vi "CalcDialogPanelBounds.vi"(8 "error in (no error)":errorcluster, 9 "Height":i32, 10 "Width":i32, 11 "Montior":i32) -> (0 "error out":errorcluster, 3 "Front Panel Window:Panel Bounds":T1)   [LabVIEW 2020, in "DP_WebView.lvclass"]
doc: "This utility will fit (resize and center) a VI (defined by the \"VI Ref\" input) about the all of the Front Panel object. It will add a border defined by border spacing in units of pixels. If no VI Reference is passed in, it will operate on the calling VI."
uses:
  DP_WebView.lvclass
  <vilib>/Utility/miscctls.llb/LVRectTypeDef.ctl
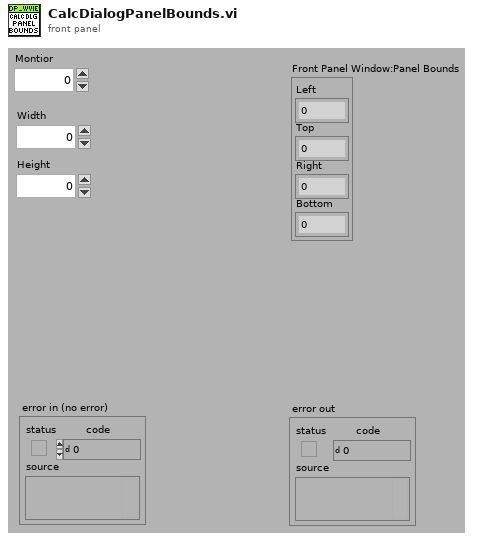
[diagram p1: front panel]
types:
  T1 = typedef "LVRectTypeDef.ctl" = cluster{"Left":i16, "Top":i16, "Right":i16, "Bottom":i16}
  T2 = typedef "LVAllMonitorsDisplayTypeDef.ctl" = cluster{"Bounds":cluster{"Left":i16, "Top":i16, "Right":i16, "Bottom":i16}, "Depth":i16}[]
  T3 = cluster{"Bounds":cluster{"Left":i16, "Top":i16, "Right":i16, "Bottom":i16}, "Depth":i16}
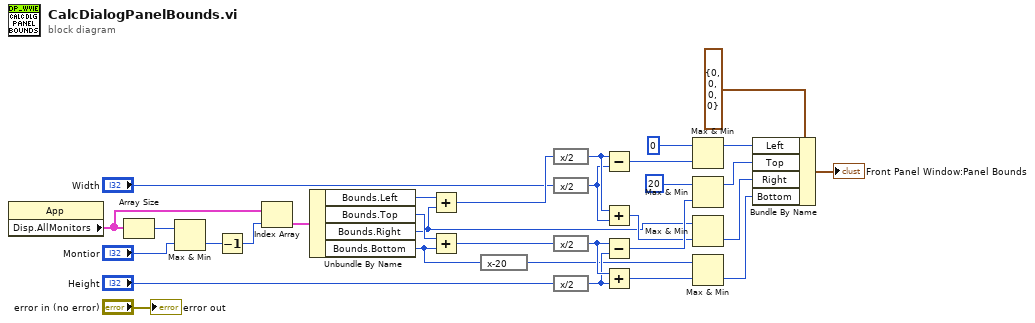
[diagram p0: block diagram]
diagram:
  n1 = property class="App"() -> ("Disp.AllMonitors"=w15:T2)  [unwired: 2 in, 2 out]
  n2 = Array Size(array=w15) -> (size(s)=w14:i32)
  n3 = Max & Min(x=w14, y="Montior") -> (min(x,y)=w12:i32)  [unwired: 1 out]
  n4 = Decrement(x=w12) -> (x-1=w16:i32)
  n5 = Index Array(array=w15, index=w16) -> (element=w30:T3)
  n6 = Unbundle By Name(w30) -> ("Bounds.Left"=w29:i16, "Bounds.Top"=w26:i16, "Bounds.Right"=w4:i16, "Bounds.Bottom"=w3:i16)
  n7 = Add(x=w29, y=w4) -> (x+y=w28:i16)
  n8 = Add(x=w26, y=w3) -> (x+y=w27:i16)
  n9 = expression code="x-20"(w3) -> (w2:i16)
  n10 = expression code="x/2"(w28) -> (w22:i16)
  n11 = expression code="x/2"("Width") -> (w21:i32)
  n12 = expression code="x/2"(w27) -> (w19:i16)
  n13 = expression code="x/2"("Height") -> (w18:i32)
  n14 = Subtract(x=w22, y=w21) -> (x-y=w20:i32)
  n15 = Add(x=w22, y=w21) -> (x+y=w8:i32)
  n16 = Subtract(x=w19, y=w18) -> (x-y=w17:i32)
  n17 = Add(x=w19, y=w18) -> (x+y=w6:i32)
  n18 = Max & Min(x=0, y=w20) -> (max(x,y)=w10:i32)  [unwired: 1 out]
  n19 = Max & Min(x=20, y=w17) -> (max(x,y)=w9:i32)  [unwired: 1 out]
  n20 = Max & Min(x=w4, y=w8) -> (min(x,y)=w7:i32)  [unwired: 1 out]
  n21 = Max & Min(x=w2, y=w6) -> (min(x,y)=w5:i32)  [unwired: 1 out]
  n22 = Bundle By Name(cluster=T1 {"Left"=0, "Top"=0, "Right"=0, "Bottom"=0} ("input cluster"), "Left"=w10, "Top"=w9, "Right"=w7, "Bottom"=w5) -> (→"Front Panel Window:Panel Bounds":T1)
  "error out" <- "error in (no error)"
